vi "String Get Words.vi"(11 "input string":string="This is a test string.") -> (3 "words":string[](array[string]))   [LabVIEW 2013, in "C Header Generator.lvlib"]
uses:
  C Header Generator.lvlib
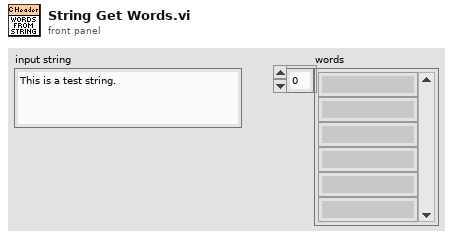
[diagram p1: front panel]
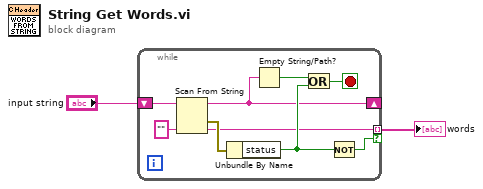
[diagram p0: block diagram]
diagram:
  n1 = while {
    tunnel: [w3] -> w1 mode=indexing if=w8
    shift-right: [w4] -> _
    shift-left: "input string" -> [w10]
    stop <- w5 stop-if-true
    n2 = Scan From String(input string=w10, default 1="") -> (remaining string=w4:string, error out=w9:errorcluster, output 1=w3:string)  [unwired: 3 in, 1 out]
    n3 = Unbundle By Name(w9) -> ("status"=w6:bool)
    n4 = Empty String/Path?(string/path=w4) -> (empty?=w7:bool)
    n5 = Or(x=w7, y=w6) -> (x .or. y?=w5:bool)
    n6 = Not(x=w6) -> (.not. x?=w8:bool)
  }
  "words" <- w1
